vi "main.vi"() -> ()   [LabVIEW 2011]
panel:
  out "path":path
  out "passYeild":dbl=0.98
  out "DB":T1={"Server"="172.20.23.107", "DB"="MESDatacenter", "PSW"="data'songyy", "User"="sa"}
  out "DB2":T1={"Server"="172.20.23.107", "DB"="HTPSDB", "PSW"="data'songyy", "User"="sa"}
  out "uploadpath":path=path "d:/xmlconvert/upload"
  out "temppath":path=path "d:/xmlconvert/temp"
  out "successpath":path=path "d:/xmlconvert/success"
  out "failpath":path=path "d:/xmlconvert/fail"
  out "path":string="D:\\testzip"
  out "timeout":i32=10
  out "filter":string="*.zip"
  in  "start":bool caption="停止"
  in  "stop":bool caption="停止"
  out "状态:":string
  in  "exit":bool caption="停止"
  # "华为异步XML生成器"
  # "Ver:1.00        20181029"
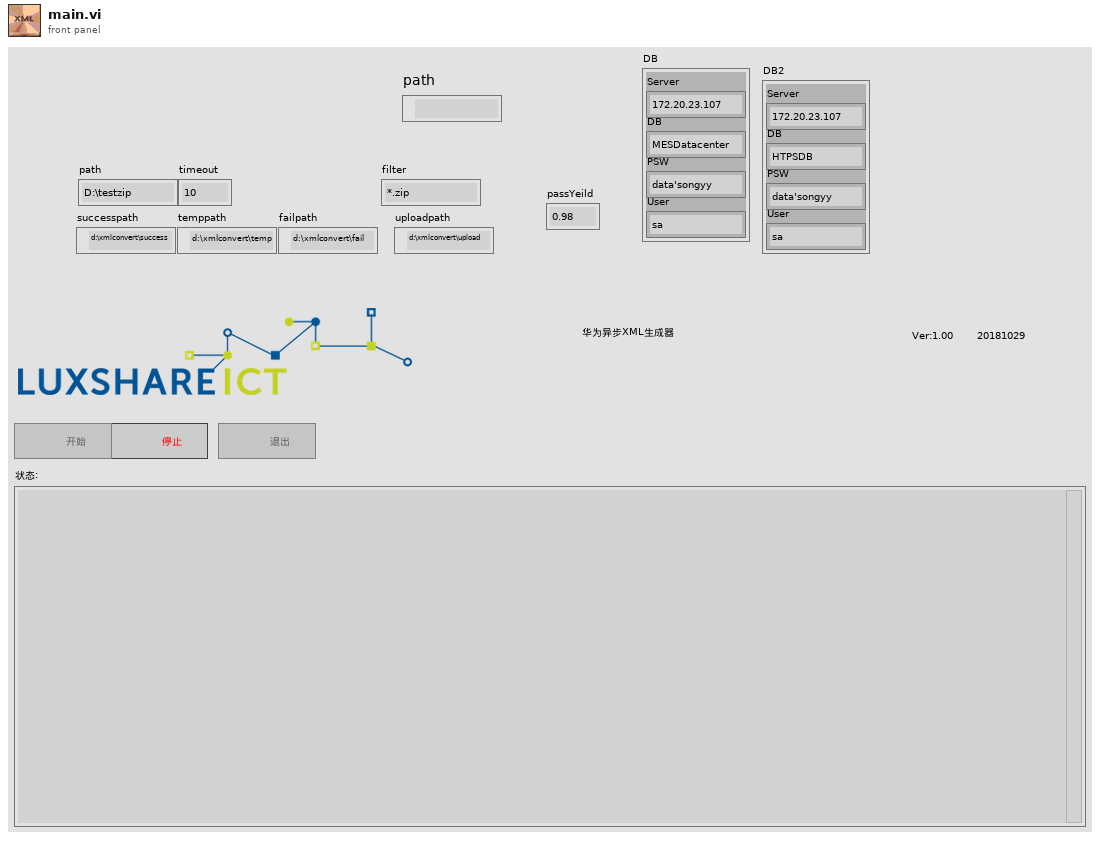
[diagram p1: front panel]
types:
  T1 = cluster{"Server":string, "DB":string, "PSW":string, "User":string}
  T2 = enum8{"Enabled", "Disabled", "Disabled and Grayed Out"}
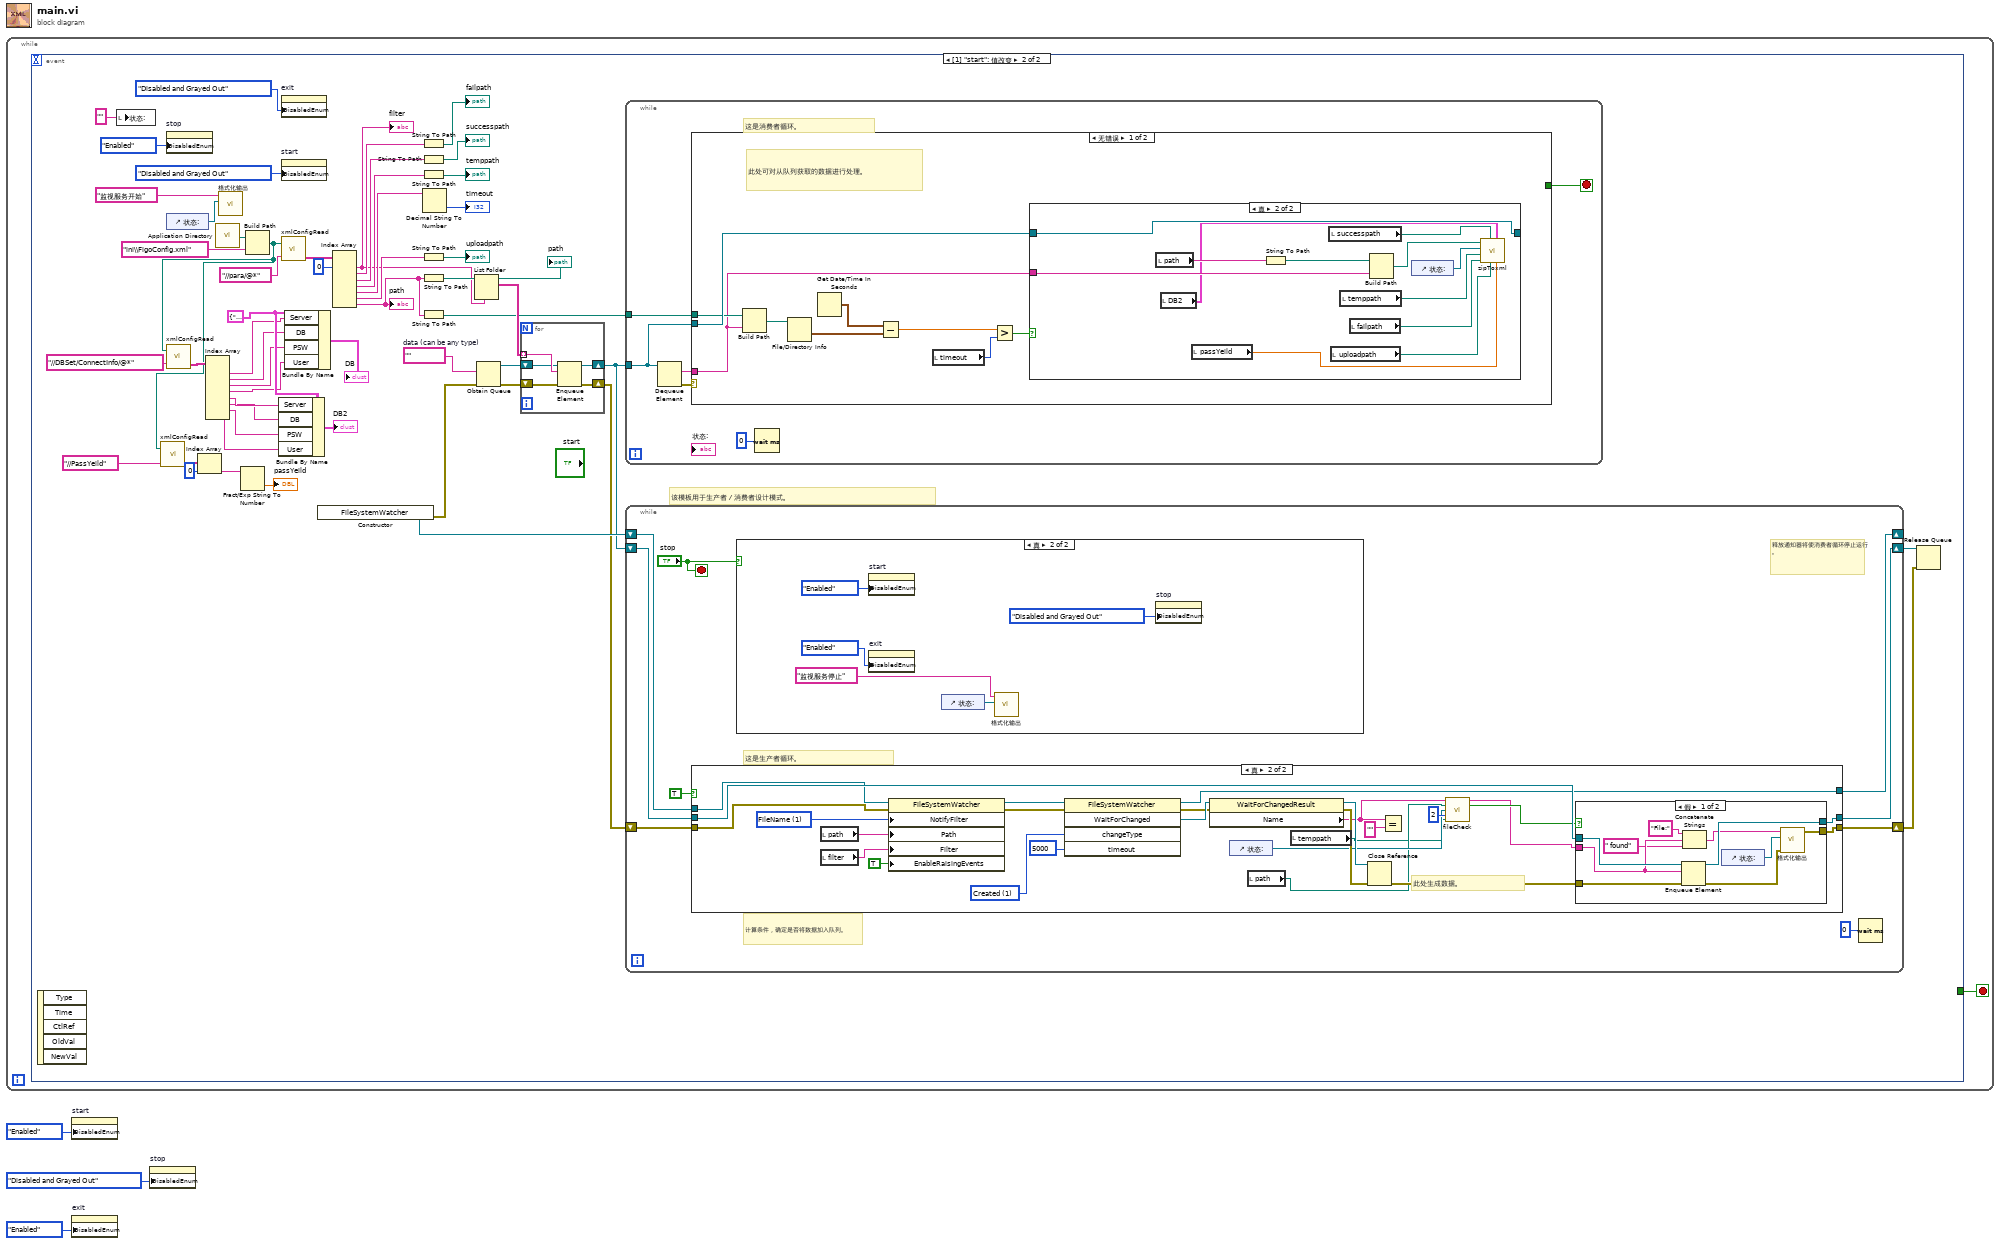
[diagram p0: block diagram]
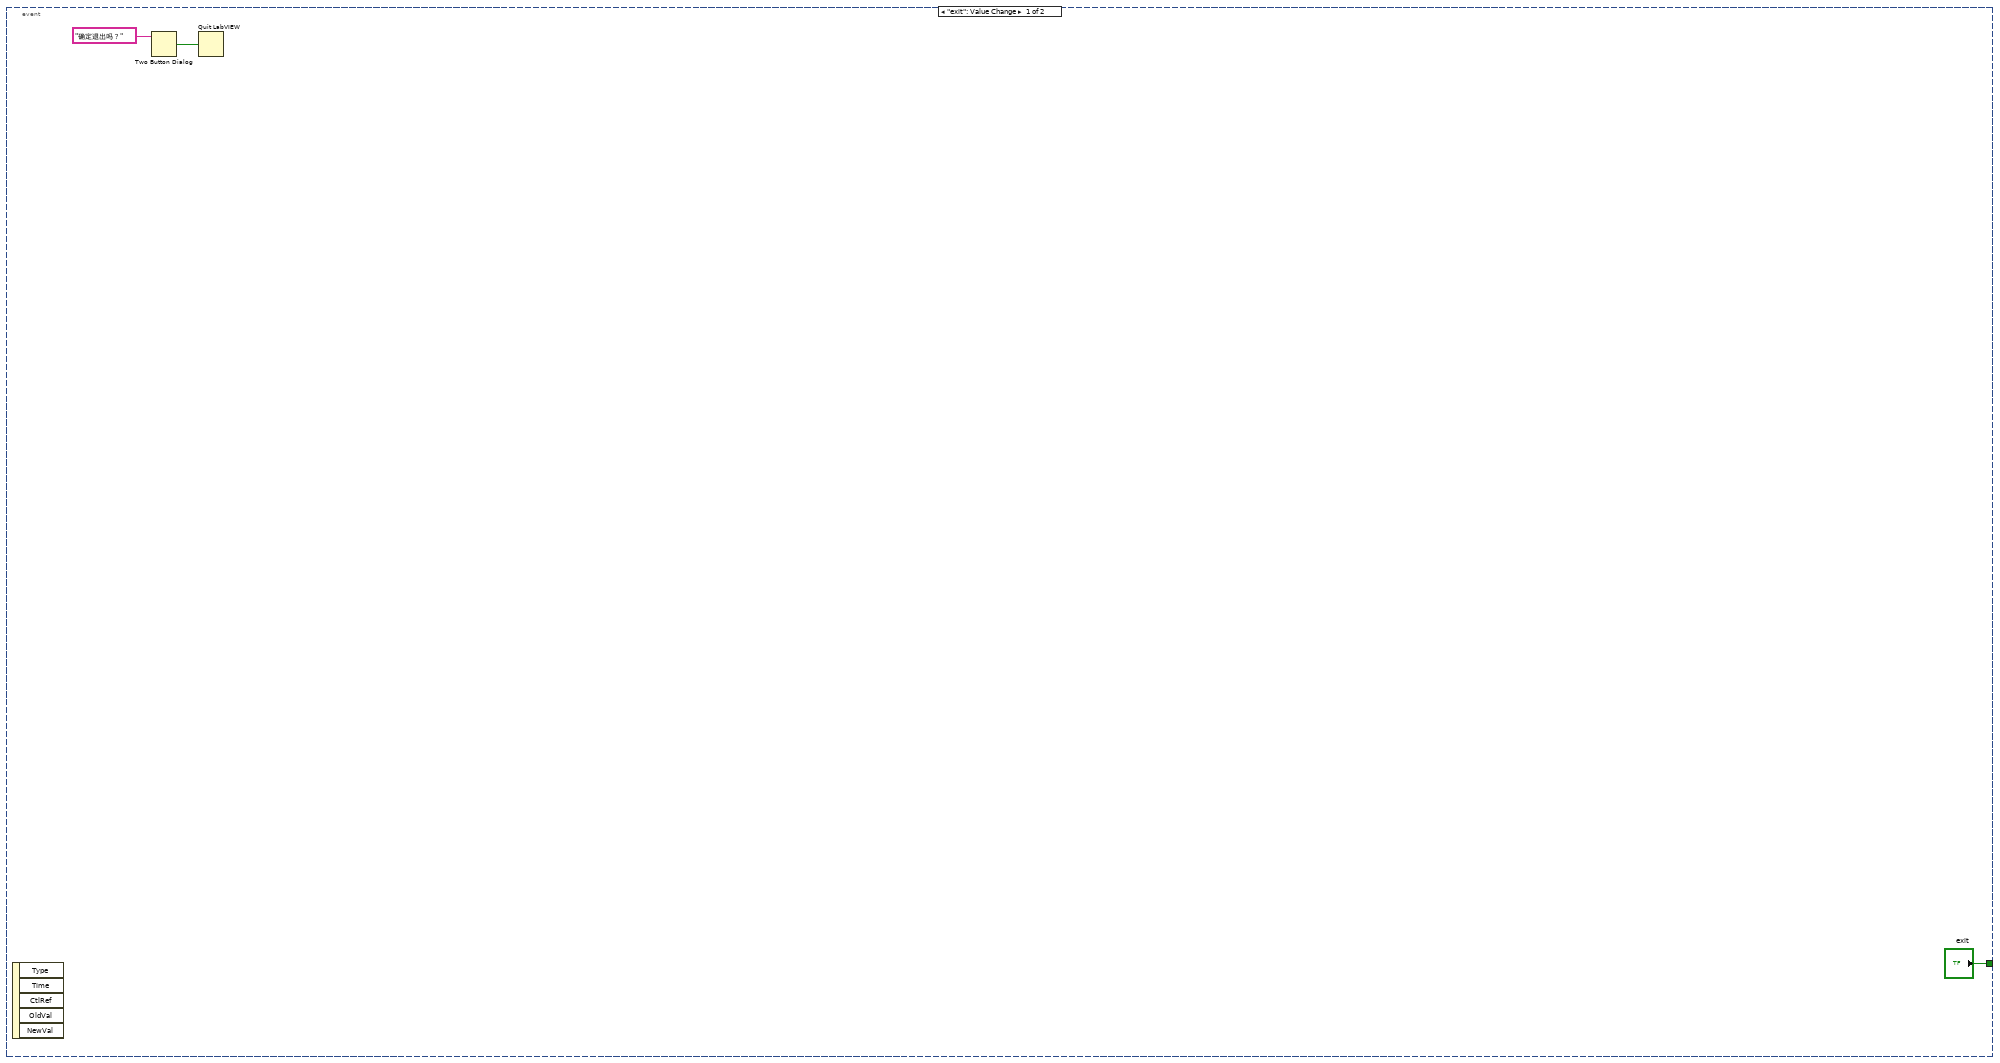
[diagram p2: hidden frame]
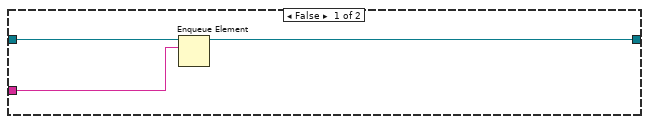
[diagram p3: hidden frame]
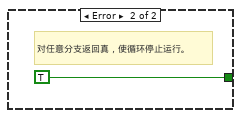
[diagram p4: hidden frame]
diagram:
  n1 = while {
    stop <- w4 stop-if-true
    n2 = event shown="[1] \"start\": 值改变" {
      selector: _ -> [_ _]
      dyn-events: _ -> [_ _]
      timeout: _ -> [_ _]
      tunnel: ["exit" _] -> w4
      event "exit": Value Change {
        n3 = event-data() -> ()  [unwired: 1 in, 5 out]
        n4 = Two Button Dialog(message="确定退出吗？" ("消息")) -> (T button?=w5:bool)  [unwired: 2 in]
        n5 = Quit LabVIEW(quit? (T)=w5) -> ()
      }
      event "start": Value Change {
        w24 = T1 {"Server"="", "DB"="", "PSW"="", "User"=""} ("DBSet")
        w59 = ""  # data (can be any type)
        # "该模板用于生产者／消费者设计模式。"
        n6 = event-data() -> ()  [unwired: 1 in, 5 out]
        n7 = local write "状态:"("" ("增加的文件")) -> ()
        n8 = property on="stop" class="Bool"("DisabledEnum"=T2."Enabled" ("禁用")) -> ()  [unwired: 2 in, 2 out]
        n9 = control-ref of="状态:"() -> (w50:refnum<vi>)
        n10 = call <vilib>:"Application Directory.vi"() -> ("Application Directory"=w47:path)
        n11 = call "格式化输出.vi"("字符串引用"=w50, "字符串"="监视服务开始") -> ()  [unwired: 9 in, 1 out]
        n12 = Build Path(base path=w47, name or relative path="ini\\FigoConfig.xml" ("名称或相对路径")) -> (appended path=w12:path)
        n13 = call "xmlConfigRead.vi"("path to XML document"=w12, "XPath expression"="//PassYeild") -> ("OutParaArray"=w11:string[])  [unwired: 2 out]
        n14 = call "xmlConfigRead.vi"("path to XML document"=w12, "XPath expression"="//DBSet/ConnectInfo/@*") -> ("OutParaArray"=w25:string[])  [unwired: 2 out]
        n15 = Index Array(array=w11, index=0 ("索引")) -> (element=w9:string)
        n16 = Index Array(array=w25) -> (element #1=w23:string, element #2=w22:string, element #3=w21:string, element #4=w20:string, element #5=w19:string, element #6=w18:string, element #7=w17:string, element #8=w16:string)  [unwired: 8 in]
        n17 = Fract/Exp String To Number(string=w9) -> (number=→"passYeild":dbl)  [unwired: 3 in, 1 out]
        n18 = Bundle By Name(cluster=w24, "Server"=w19, "DB"=w18, "PSW"=w17, "User"=w16) -> (→"DB2":T1)
        n19 = property on="exit" class="Bool"("DisabledEnum"=T2."Disabled and Grayed Out" ("禁用")) -> ()  [unwired: 2 in, 2 out]
        n20 = property on="start" class="Bool"("DisabledEnum"=T2."Disabled and Grayed Out" ("禁用")) -> ()  [unwired: 2 in, 2 out]
        n21 = call "xmlConfigRead.vi"("path to XML document"=w12, "XPath expression"="//para/@*") -> ("OutParaArray"=w44:string[])  [unwired: 2 out]
        n22 = Bundle By Name(cluster=w24, "Server"=w23, "DB"=w22, "PSW"=w21, "User"=w20) -> (→"DB":T1)
        n23 = constructor class="FileSystemWatcher"() -> (reference out=w58:refnum<k24>, error out=w57:errorcluster)  [unwired: 3 in, 1 out]
        n24 = Index Array(array=w44, index #1=0 ("索引")) -> (element #1=w27:string, element #2=w39:string, element #3=w37:string, element #4=w34:string, element #5=w35:string, element #6=w32:string, element #7=w28:string)  [unwired: 6 in]
        "filter" <- w27
        "path" <- w28
        n25 = String To Path(string=w39) -> (path=→"failpath":path)
        n26 = String To Path(string=w37) -> (path=→"successpath":path)
        n27 = String To Path(string=w34) -> (path=→"temppath":path)
        n28 = String To Path(string=w32) -> (path=→"uploadpath":path)
        n29 = String To Path(string=w28) -> (path=w56:path)
        "path" <- w56
        n30 = String To Path(string=w28) -> (path=w41:path)
        n31 = Decimal String To Number(string=w35) -> (number=→"timeout":i32)  [unwired: 2 in, 1 out]
        n32 = List Folder(path=w56, pattern=w27) -> (filenames=w55:string[])  [unwired: 2 in, 3 out]
        n33 = Obtain Queue(element data type=w59, error in (no error)=w57) -> (queue out=w54:refnum<queue>, error out=w53:errorcluster)  [unwired: 3 in, 1 out]
        n34 = for {
          tunnel: w55 -> [w66] mode=indexing
          shift-right: [w64] -> w51
          shift-left: w54 -> [w65]
          shift-right: [w62] -> w52
          shift-left: w53 -> [w63]
          n35 = Enqueue Element(queue=w65, element=w66, error in (no error)=w63) -> (queue out=w64:refnum<queue>, error out=w62:errorcluster)  [unwired: 1 in, 1 out]
        }
        n36 = while {
          tunnel: w51 -> [w69]
          tunnel: w41 -> [w67]
          stop <- w70 stop-if-true
          # "这是消费者循环。"
          n37 = Dequeue Element(queue=w69) -> (element=w71:string, error out=w72:errorcluster)  [unwired: 2 in, 2 out]
          n38 = case shown="无错误" w72 {
            tunnel: w71 -> [w75 _]
            tunnel: [_ TRUE] -> w70
            tunnel: w69 -> [w77 _]
            tunnel: w67 -> [w76 _]
            frame No Error {
              # "此处可对从队列获取的数据进行处理。"
              n39 = Build Path(base path=w76, name or relative path=w75) -> (appended path=w74:path)
              n40 = File/Directory Info(path=w74) -> (last mod=w79:timestamp)  [unwired: 1 in, 6 out]
              n41 = Get Date/Time In Seconds() -> (seconds since 1Jan1904=w80:timestamp)
              n42 = Subtract(x=w80, y=w79) -> (x-y=w81:dbl)
              n43 = local read "timeout"() -> (w73:i32)
              n44 = Greater?(x=w81, y=w73) -> (0:w78:bool)
              n45 = case shown="真" w78 {
                tunnel: w77 -> [w84 w96]
                tunnel: w75 -> [w83 w93]
                tunnel: [w82 w96] -> _
                frame False {
                  n46 = Enqueue Element(queue=w84, element=w83) -> (queue out=w82:refnum<queue>)  [unwired: 2 in, 2 out]
                }
                frame True {
                  n47 = local read "path"() -> (w91:string)
                  n48 = local read "DB2"() -> (w86:T1)
                  n49 = local read "passYeild"() -> (w85:dbl)
                  n50 = String To Path(string=w91) -> (path=w95:path)
                  n51 = local read "successpath"() -> (w88:path)
                  n52 = local read "uploadpath"() -> (w87:path)
                  n53 = local read "temppath"() -> (w90:path)
                  n54 = local read "failpath"() -> (w89:path)
                  n55 = Build Path(base path=w95, name or relative path=w93) -> (appended path=w94:path)
                  n56 = control-ref of="状态:"() -> (w92:refnum<vi>)
                  n57 = call "zipToxml.vi"("passYield"=w85, "DBSet"=w86, "uploadPath"=w87, "successxmlpath"=w88, "转换失败路径"=w89, "目标路径"=w90, "status msg ref"=w92, "path"=w94) -> ()  [unwired: 4 in]
                }
              }
            }
            frame Error {
              # "对任意分支返回真，使循环停止运行。"
            }
          }
          n58 = Wait (ms)(milliseconds to wait=u32 0 ("等待时间（毫秒）")) -> ()  [unwired: 1 out]
        }
        n59 = while {
          shift-right: [w103] -> w60
          shift-left: w52 -> [w104]
          shift-right: [w105] -> w61
          shift-left: w51 -> [w106]
          shift-right: [w100] -> _
          shift-left: w58 -> [w101]
          stop <- "stop" stop-if-true
          # "释放通知器将使消费者循环停止运行。"
          # "计算条件，确定是否将数据加入队列。"
          # "这是生产者循环。"
          n60 = case shown="真" TRUE ("Case Constant\n(See Context Help)") {
            tunnel: w106 -> [w114 w134]
            tunnel: [w114 w132] -> w105
            tunnel: w104 -> [w113 w125]
            tunnel: [w113 w133] -> w103
            tunnel: w101 -> [w112 w127]
            tunnel: [w112 w126] -> w100
            frame False {
            }
            frame True {
              w138 = 1 items=["Created"=1, "Deleted"=2, "Changed"=4, "Renamed"=8, "All"=15] ("changeType")
              w140 = 1 items=["FileName"=1, "DirectoryName"=2, "Attributes"=4, "Size"=8, "LastWrite"=16, "LastAccess"=32, "CreationTime"=64, "Security"=256] ("NotifyFilter")
              # "此处生成数据。"
              n61 = local read "path"() -> (w123:string)
              n62 = local read "filter"() -> (w122:string)
              n63 = property class="FileSystemWatcher"(reference=w127, error in=w125, "NotifyFilter"=w140, "Path"=w123, "Filter"=w122, "EnableRaisingEvents"=TRUE) -> (reference out=w139:refnum<k24>, error out=w131:errorcluster)
              n64 = invoke class="FileSystemWatcher" method="WaitForChanged"(reference=w139, error in=w131, "changeType"=w138, "timeout"=5000) -> (reference out=w126:refnum<k24>, error out=w130:errorcluster, "WaitForChanged"=w136:refnum<k24>)  [unwired: 1 in, 2 out]
              n65 = property class="WaitForChangedResult"(reference=w136, error in=w130) -> (reference out=w129:refnum<k24>, error out=w128:errorcluster, "Name"=w121:string)
              n66 = control-ref of="状态:"() -> (w117:refnum<vi>)
              n67 = local read "path"() -> (w116:path)
              n68 = local read "temppath"() -> (w115:path)
              n69 = Close Reference(reference=w129, error in (no error)=w128) -> (error out=w124:errorcluster)
              n70 = Equal?(x=w121, y="") -> ()  [unwired: 1 out]
              n71 = call "fileCheck.vi"("fileName"=w121, "netPath"=w116, "status"=w117, "testCount"=2, "basicPath"=w115) -> ("fileName Out"=w119:string, "布尔"=w120:bool)  [unwired: 9 in]
              n72 = case shown="假" w120 {
                tunnel: w134 -> [w151 w152]
                tunnel: w124 -> [w150 w153]
                tunnel: [w143 w153] -> w133
                tunnel: [w149 w152] -> w132
                tunnel: w119 -> [w147 _]
                frame False {
                  n73 = Enqueue Element(queue=w151, element=w147, error in (no error)=w150) -> (queue out=w149:refnum<queue>, error out=w144:errorcluster)  [unwired: 1 in, 1 out]
                  n74 = Concatenate Strings("File:" ("字符串"), w147, " found" ("字符串")) -> (w145:string)
                  n75 = control-ref of="状态:"() -> (w142:refnum<vi>)
                  n76 = call "格式化输出.vi"("错误输入（无错误）"=w144, "字符串引用"=w142, "字符串"=w145) -> ("错误输出"=w143:errorcluster)  [unwired: 8 in]
                }
                frame True {
                }
              }
            }
          }
          n77 = case shown="真" "stop" {
            frame False {
            }
            frame True {
              n78 = property on="start" class="Bool"("DisabledEnum"=T2."Enabled" ("禁用")) -> ()  [unwired: 2 in, 2 out]
              n79 = property on="exit" class="Bool"("DisabledEnum"=T2."Enabled" ("禁用")) -> ()  [unwired: 2 in, 2 out]
              n80 = control-ref of="状态:"() -> (w111:refnum<vi>)
              n81 = call "格式化输出.vi"("字符串引用"=w111, "字符串"="监视服务停止") -> ()  [unwired: 9 in, 1 out]
              n82 = property on="stop" class="Bool"("DisabledEnum"=T2."Disabled and Grayed Out" ("禁用")) -> ()  [unwired: 2 in, 2 out]
            }
          }
          n83 = Wait (ms)(milliseconds to wait=u32 0 ("等待时间（毫秒）")) -> ()  [unwired: 1 out]
        }
        n84 = Release Queue(queue=w61, error in (no error)=w60) -> ()  [unwired: 1 in, 3 out]
      }
    }
  }
  n85 = property on="start" class="Bool"("DisabledEnum"=T2."Enabled" ("禁用")) -> ()  [unwired: 2 in, 2 out]
  n86 = property on="exit" class="Bool"("DisabledEnum"=T2."Enabled" ("禁用")) -> ()  [unwired: 2 in, 2 out]
  n87 = property on="stop" class="Bool"("DisabledEnum"=T2."Disabled and Grayed Out" ("禁用")) -> ()  [unwired: 2 in, 2 out]
